vi "sub_distance_processing1.vi"(1 "Calibration":T1 {"r bias" format="%_3p"; "Ks" format="%#_3p"}, 3 "Reset RMS":bool, 5 "Output options":T2, 7 "High/low index":i32, 9 "Magnitude":dbl[](array[numeric]), 11 "Fs low":dbl=1.0, 12 "Fs":dbl, 13 "Reset":bool, 14 "Time Stamp":timestamp) -> (4 "RMS":dbl, 6 "DC":dbl, 8 "Mean level":dbl, 10 "Waveform":waveform(dbl))   [LabVIEW 2026]
uses:
  gui/output_options.ctl
  gui/coupling_selector.ctl
  calibration.ctl
  <vilib>/Analysis/3filter.llb/Filter Passband Type.ctl
  <vilib>/Analysis/baseanly.llb/IIR Cascade Filter (DBL).vi
  <vilib>/Analysis/NI_AALBase.lvlib
panel:
  # "0 = high"
  # "Demodulated magnitude (high or low)"
  # "Sample rate we are called at (low rate)"
  # "Sample rate of magnitude"
  # "This VI deals with distance processing for either high or low, separately so that we can use re-entrant filter VIs"
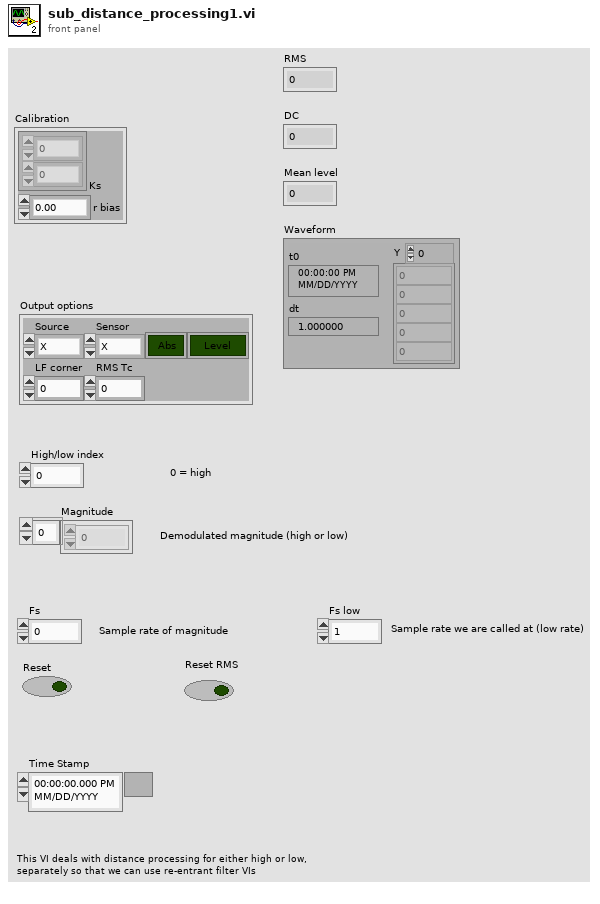
[diagram p1: front panel]
types:
  T1 = typedef "calibration.ctl" = cluster{"Ks":dbl[], "r bias":dbl}
  T2 = typedef "output_options.ctl" = cluster{"Source":T3, "Sensor":T3, "Sense":bool, "Distance":bool, "LF corner":dbl, "RMS Tc":dbl}
  T3 = typedef "coupling_selector.ctl" = enum16{"X", "Y", "Z", "Vector"}
  T4 = cluster{"filter structure":enum32{"IIR 2nd Order", "IIR 4th Order"}, "Reverse Coefficients":dbl[], "Forward Coefficients":dbl[]}
  T5 = typedef "NI_AALBase.lvlib/Filter Passband Type.ctl" = enum32{"Lowpass", "Highpass", "Bandpass", "Bandstop"}
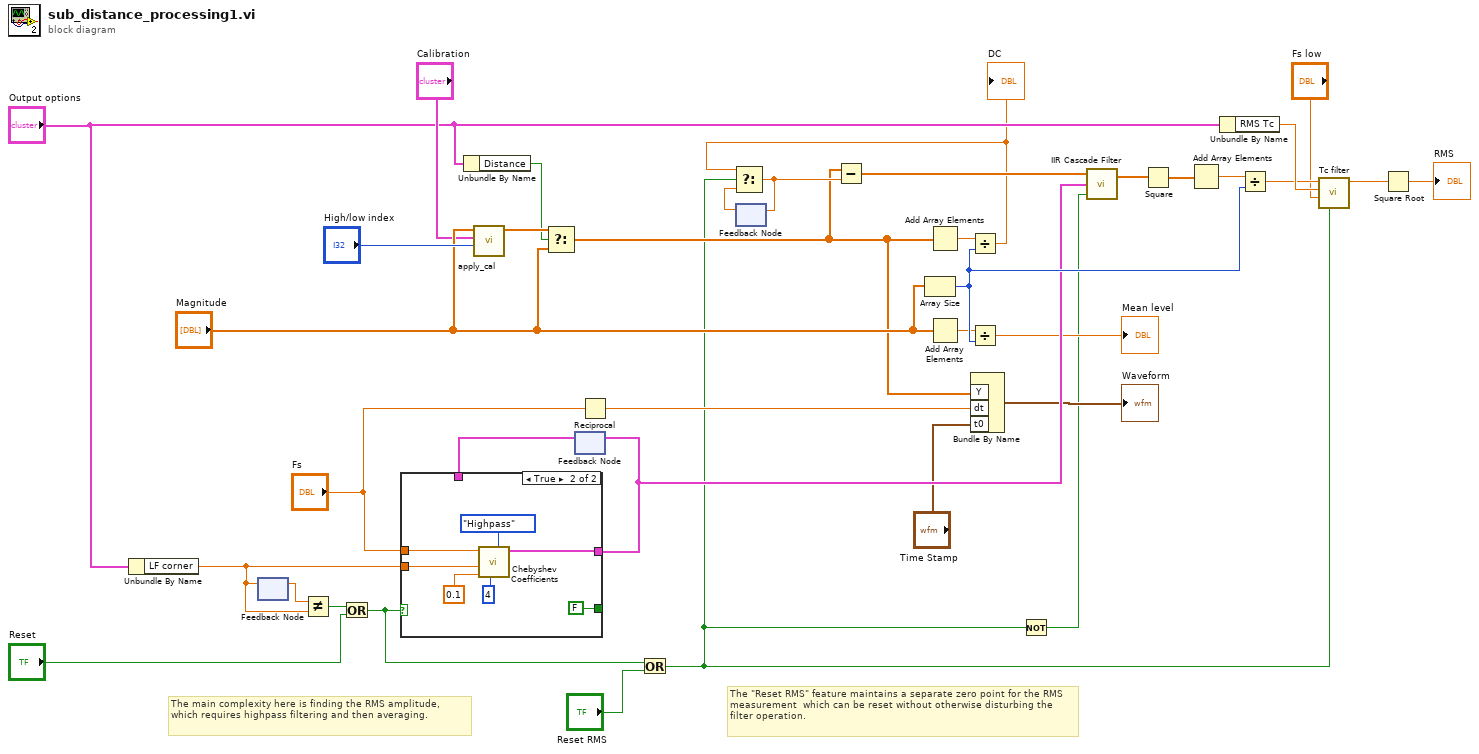
[diagram p0: block diagram]
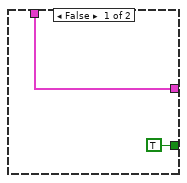
[diagram p2: hidden frame]
diagram:
  # "The \"Reset RMS\" feature maintains a separate zero point for the RMS measurement  which can be reset without otherwise disturbing the filter operation."
  # "The main complexity here is finding the RMS amplitude, which requires highpass filtering and then averaging."
  n1 = Unbundle By Name("Output options") -> ("LF corner"=w10:dbl)
  n2 = feedback #1() -> (w27:dbl)  [unwired: 1 in]
  n3 = feedback-in #1(w10) -> ()
  n4 = Not Equal?(x=w27, y=w10) -> (x != y?=w28:bool)
  n5 = Or(x=w28, y="Reset") -> (x .or. y?=w1:bool)
  n6 = Unbundle By Name("Output options") -> ("Distance"=w14:bool)
  n7 = call "apply_cal.vi"("High/low index"="High/low index", "Calibration"="Calibration", "V"="Magnitude") -> ("r"=w22:dbl[])  [unwired: 8 in]
  n8 = Select(t=w22, s=w14, f="Magnitude") -> (s? t:f=w5:dbl[])
  n9 = feedback #2() -> (w29:T4)  [unwired: 1 in]
  n10 = case shown="True" w1 {
    tunnel: w10 -> [_ w42]
    tunnel: [w39 w44] -> w31
    tunnel: w29 -> [w39 _]
    tunnel: "Fs" -> [_ w43]
    tunnel: [TRUE ("Reset") FALSE ("Reset")] -> _
    frame False {
    }
    frame True {
      n11 = call <vilib>:"Chebyshev Coefficients.vi"("order"=4, "filter type"=Filter_Passband_Type."Highpass", "ripple(dB)"=0.1, "low cutoff freq: fl"=w42, "sampling freq: fs"=w43) -> ("IIR Filter Cluster"=w44:T4)  [unwired: 5 in, 1 out]
    }
  }
  n12 = feedback-in #2(w31) -> ()
  n13 = Reciprocal(x="Fs") -> (1/x=w30:dbl)
  n14 = Or(x=w1, y="Reset RMS") -> (x .or. y?=w3:bool)
  n15 = feedback #3() -> (w7:dbl)  [unwired: 1 in]
  n16 = Array Size(array="Magnitude") -> (size(s)=w34:i32)
  n17 = Add Array Elements(numeric array=w5) -> (sum=w20:dbl)
  n18 = Add Array Elements(numeric array="Magnitude") -> (sum=w21:dbl)
  n19 = Divide(x=w20, y=w34) -> (x/y=w8:dbl)
  "DC" <- w8
  n20 = Select(t=w8, s=w3, f=w7) -> (s? t:f=w6:dbl)
  n21 = feedback-in #3(w6) -> ()
  n22 = Subtract(x=w5, y=w6) -> (x-y=w12:dbl[])
  n23 = Divide(x=w21, y=w34) -> (x/y=→"Mean level":dbl)
  n24 = Bundle By Name("Y"=w5, "dt"=w30, "t0"="Time Stamp") -> (→"Waveform":waveform(dbl))  [unwired: 1 in]
  n25 = Not(x=w3) -> (.not. x?=w4:bool)
  n26 = call-poly <vilib>:"IIR Cascade Filter.vi"("init/cont (init:F)"=w4, "IIR Filter Cluster"=w31, "X"=w12) -> ("Filtered X"=w13:dbl[])  [unwired: 1 out]
  n27 = Square(x=w13) -> (x^2=w32:dbl[])
  n28 = Add Array Elements(numeric array=w32) -> (sum=w33:dbl)
  n29 = Unbundle By Name("Output options") -> ("RMS Tc"=w36:dbl)
  n30 = Divide(x=w33, y=w34) -> (x/y=w35:dbl)
  n31 = call "Tc filter.vi"("Reset"=w3, "Fs"="Fs low", "Tc"=w36, "Input"=w35) -> ("Output"=w16:dbl)  [unwired: 7 in]
  n32 = Square Root(x=w16) -> (sqrt(x)=→"RMS":dbl)
